vi "variantCtrlIo.vi"(4 "isRequired (T)":bool=TRUE, 6 "menu (Get Param)":T6, 8 "error in":errorcluster, 10 "Key (use IOnode Label if empty )":string, 11 "IOnode in":T1={"ADDR"=0, "Label"="", "Type"=enum."DI", "Mode"=enum."RIO", "Value"="", "Tags"="", "calibration"=[]} {"calibration"."Y" format="%#.3f"; "calibration"."X" format="%#.3f"; "ADDR" format="%04d"}) -> (0 "error out":errorcluster, 1 "I/O names":string[](array[string]), 2 "found":bool, 3 "IOnode out":T1={"ADDR"=0, "Label"="", "Type"=enum."DI", "Mode"=enum."RIO", "Value"="", "Tags"="", "calibration"=[]} {"calibration"."Y" format="%#.3f"; "calibration"."X" format="%#.3f"; "ADDR" format="%04d"}, 5 "IO Configs List":T1[](array[typedef]) {"calibration"."Y" format="%#.3f"; "calibration"."X" format="%#.3f"; "ADDR" format="%04d"})   [LabVIEW 2024]
uses:
  controls/IONode.ctl
  controls/type.address.ctl
  controls/enum.io.type.ctl
  controls/enum.io.mode.ctl
  controls/typeXyPoint.ctl
  controls/enumVarCtrlIO.ctl
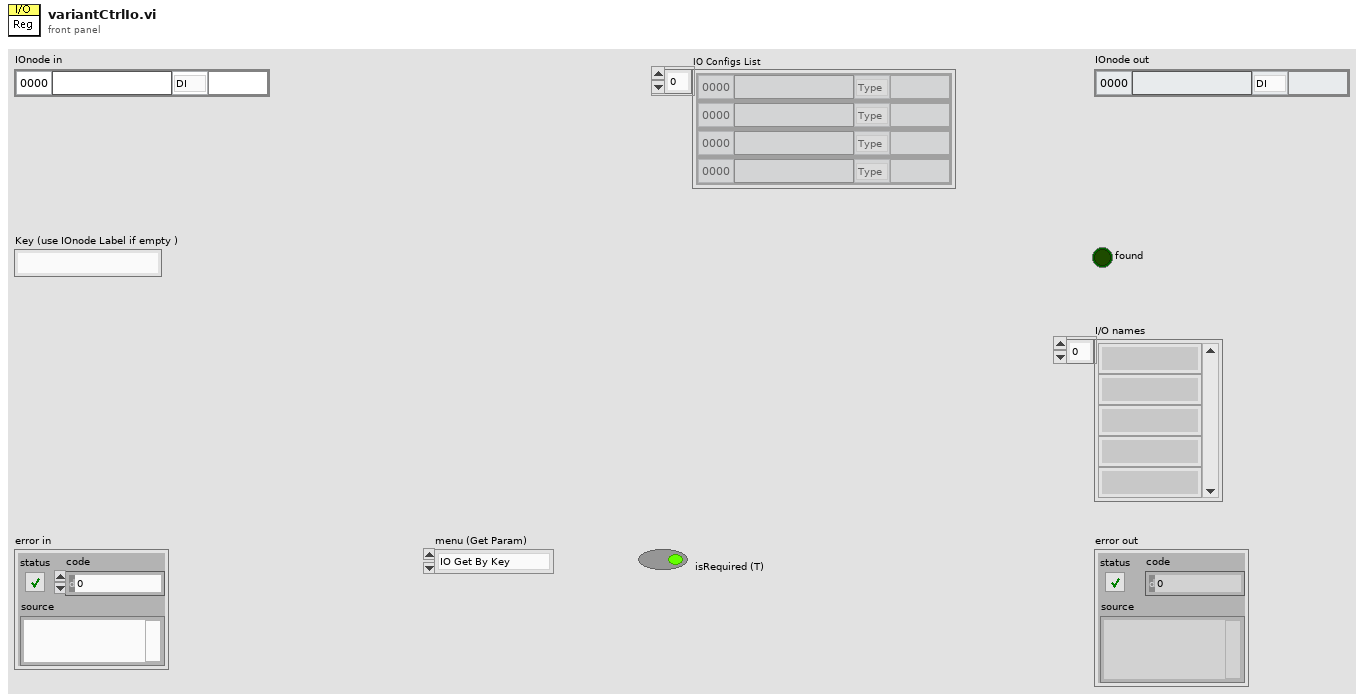
[diagram p1: front panel]
types:
  T1 = typedef "IONode.ctl" = cluster{"ADDR":T2, "Label":string, "Type":T3, "Mode":T4, "Value":string, "Tags":string, "calibration":T5[]}
  T2 = typedef "type.address.ctl" = u16
  T3 = typedef "enum.io.type.ctl" = enum16{"Type", "DI", "DO", "AI", "AO", "VL", "BUF"}
  T4 = typedef "enum.io.mode.ctl" = enum16{"Mode", "RIO", "SIM"}
  T5 = typedef "typeXyPoint.ctl" = cluster{"X":dbl, "Y":dbl}
  T6 = typedef "enumVarCtrlIO.ctl" = enum16{"IO Get By Key", "IO List Configs", "IO Add By Key", "IO Modify Value By Key", "IO Modify Calib By Key", "IO Modify ADDR By Key", "IO Modify Mode By Key", "IO Modify Type By Key", "IO Modify Name By Key", "IO Remove By Key", "IO Remove All"}
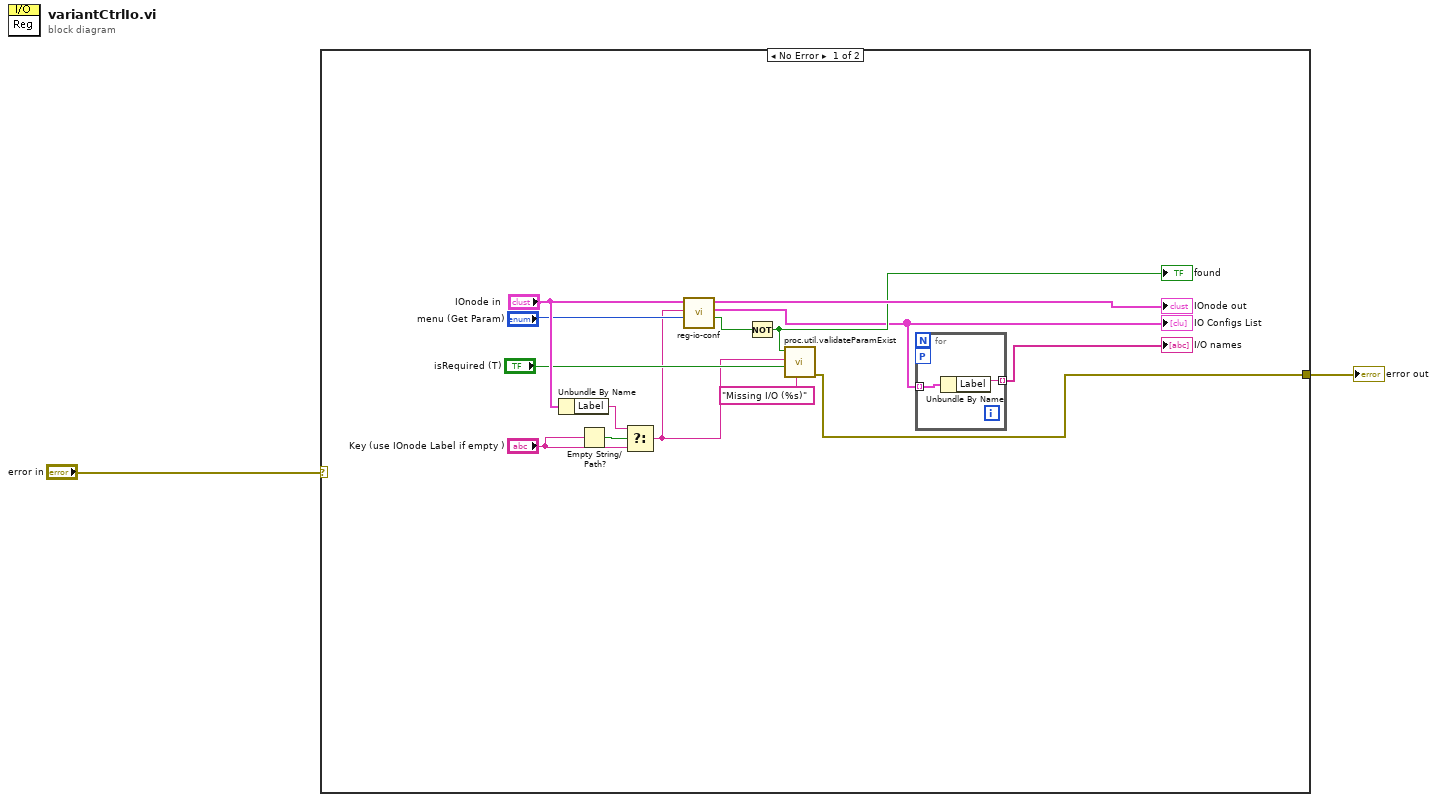
[diagram p0: block diagram]
diagram:
  n1 = case shown="No Error" "error in" {
    selector: "error in" -> [_ w19]
    tunnel: [w11 w19] -> w2
    frame No Error {
      n2 = Unbundle By Name("IOnode in") -> ("Label"=w5:string)
      n3 = Empty String/Path?(string/path="Key (use IOnode Label if empty )") -> (empty?=w6:bool)
      n4 = Select(t=w5, s=w6, f="Key (use IOnode Label if empty )") -> (s? t:f=w4:string)
      n5 = call "reg-io-conf.vi"("menu (List Configs)"="menu (Get Param)", "Key"=w4, "IO Node in"="IOnode in") -> ("Key Not Found?"=w7:bool, "List Nodes"=w9:T1[], "IO Node out"=→"IOnode out":T1)  [unwired: 6 in]
      "IO Configs List" <- w9
      n6 = Not(x=w7) -> (.not. x?=w12:bool)
      "found" <- w12
      n7 = call "proc.util.validateParamExist.vi"("format string"="Missing I/O (%s)", "isRequired"="isRequired (T)", "Param Label"=w4, "isFound"=w12) -> ("error out"=w11:errorcluster)  [unwired: 7 in]
      n8 = for {
        tunnel: w9 -> [w18] mode=indexing
        tunnel: [w17] -> w10 mode=indexing
        workers-P: _ -> [_]
        n9 = Unbundle By Name(w18) -> ("Label"=w17:string)
      }
      "I/O names" <- w10
    }
    frame Error {
    }
  }
  "error out" <- w2
